vi "SSL_CTX_use_certificate.vi"(8 "error in (no error)":errorcluster, 9 "cert path":T1, 10 "CTX":i32, 11 "path in":path) -> (0 "error out":errorcluster, 2 "CTX":i32, 3 "path out":path)   [LabVIEW 2015, in "AWS_IoT.lvlib"]
uses:
  AWS_IoT.lvlib
  Controls/certs.ctl
panel:
  out "return type 5":i32
  out "return type 2":i32
  out "return type":i32
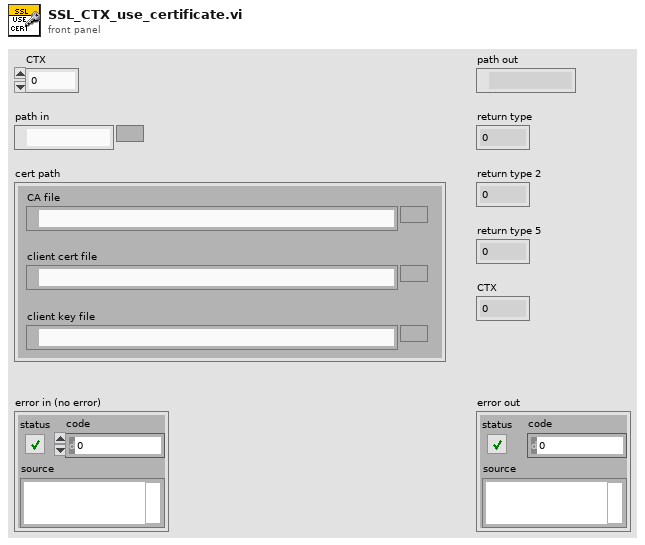
[diagram p1: front panel]
types:
  T1 = typedef "AWS_IoT.lvlib/certs.ctl" = cluster{"client cert file":path, "CA file":path, "client key file":path}
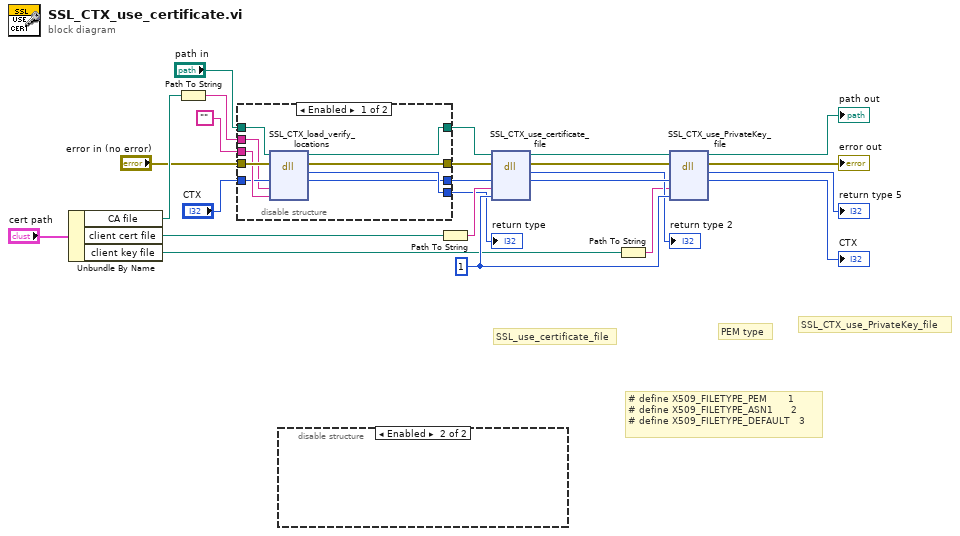
[diagram p0: block diagram]
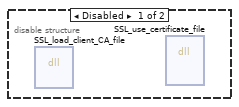
[diagram p2: hidden frame]
diagram:
  w21 = 1 ("type")
  # "# define X509_FILETYPE_PEM       1\n# define X509_FILETYPE_ASN1      2\n# define X509_FILETYPE_DEFAULT   3"
  # "SSL_CTX_use_PrivateKey_file"
  # "PEM type"
  # "SSL_use_certificate_file"
  n1 = Unbundle By Name("cert path") -> ("CA file"=w7:path, "client cert file"=w8:path, "client key file"=w9:path)
  n2 = Path To String(path=w7) -> (string=w5:string)
  n3 = disable-structure shown="Enabled" {
    disable-tunnel: "path in" -> [w33 w36]
    disable-tunnel: "error in (no error)" -> [w32 w35]
    disable-tunnel: "" ("CApath") -> [w31 _]
    disable-tunnel: "CTX" -> [w30 w34]
    disable-tunnel: w5 -> [w29 _]
    disable-tunnel: [w28 _] -> w10
    disable-tunnel: [w27 w36] -> w13
    disable-tunnel: [w26 w35] -> w15
    disable-tunnel: [w25 w34] -> w19
    frame Enabled {
      n4 = dll-call lib="NIssleay32.*" fn="SSL_CTX_load_verify_locations"(path in=w33, error in=w32, "CTX"=w30, "CAfile"=w29, "CApath"=w31) -> (path out=w27:path, error out=w26:errorcluster, "return type"=w28:i32, "CTX"=w25:i32)  [unwired: 3 in]
    }
    frame Disabled {
    }
  }
  "return type" <- w10
  n5 = disable-structure shown="Enabled" {
    frame Disabled {
      n6 = dll-call lib="NIssleay32.*" fn="SSL_load_client_CA_file"() -> ()  [unwired: 8 in, 2 out]
      n7 = dll-call lib="NIssleay32.*" fn="SSL_use_certificate_file"() -> ()  [unwired: 10 in, 2 out]
    }
    frame Enabled {
    }
  }
  n8 = Path To String(path=w8) -> (string=w20:string)
  n9 = dll-call lib="NIssleay32.*" fn="SSL_CTX_use_certificate_file"(path in=w13, error in=w15, "CTX"=w19, "keyfile"=w20, "type"=w21) -> (path out=w14:path, error out=w16:errorcluster, "return type"=→"return type 2":i32, "CTX"=w18:i32)  [unwired: 3 in]
  n10 = Path To String(path=w9) -> (string=w12:string)
  n11 = dll-call lib="NIssleay32.*" fn="SSL_CTX_use_PrivateKey_file"(path in=w14, error in=w16, "CTX"=w18, "keyfile"=w12, "type"=w21) -> (path out=→"path out":path, error out=→"error out":errorcluster, "return type"=→"return type 5":i32, "CTX"=→"CTX":i32)  [unwired: 3 in]
